vi "Register gRPC Messages.vi"(8 "error in (no error)":errorcluster, 11 "Template Server in":refnum<class "HVC5.lvclass">) -> (0 "error out":errorcluster, 3 "Template Server out":refnum<class "HVC5.lvclass">)   [LabVIEW 2019, in "HVC5.lvlib" / "HVC5.lvclass"]
uses:
  HVC5.lvclass
  gRPC lvSupport/Server API/typeDefs/Message Metadata.ctl
  gRPC lvSupport/Server API/typeDefs/Message Element Metadata.ctl
  gRPC lvSupport/Server API/typeDefs/Message Element Type.ctl
  HVC5.lvclass/HVC5.ctl
  gRPC lvSupport/gprc-lvsupport.lvlib
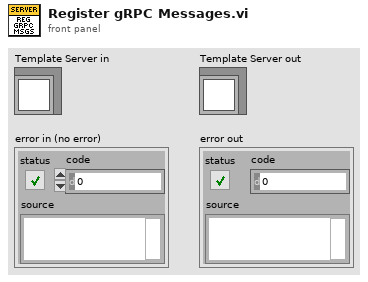
[diagram p1: front panel]
types:
  T1 = typedef "HVC5.lvlib/gprc-lvsupport.lvlib/Message Metadata.ctl" = cluster{"Name":string, "Elements":T2[]}
  T2 = typedef "HVC5.lvlib/gprc-lvsupport.lvlib/Message Element Metadata.ctl" = cluster{"Embedded Message Name":string, "Protobuf Index":i32, "MessageElementType":T3, "Repeated":bool}
  T3 = typedef "HVC5.lvlib/gprc-lvsupport.lvlib/Message Element Type.ctl" = enum32{"Int32Value", "FloatValue", "DoubleValue", "BoolValue", "StringValue", "MessageValue", "Int64Value", "UInt32Value", "UInt64Value", "EnumValue"}
  T4 = typedef "HVC5.lvlib/gprc-lvsupport.lvlib/grpcId.ctl" = u64
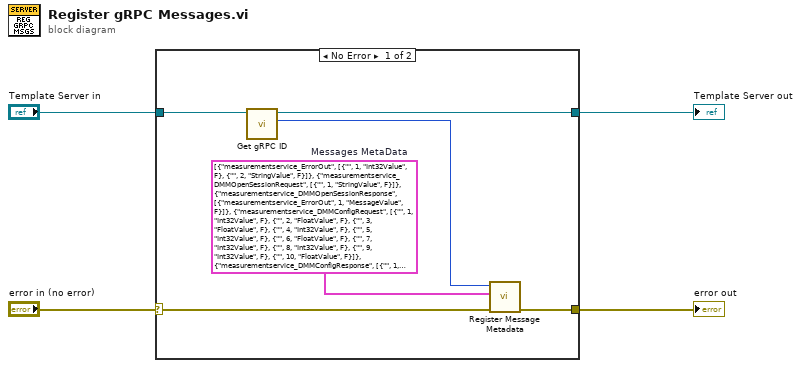
[diagram p0: block diagram]
diagram:
  n1 = case shown="No Error" "error in (no error)" {
    selector: "error in (no error)" -> [w5 w12]
    tunnel: [w10 w11] -> w4
    tunnel: [w9 w12] -> w3
    tunnel: "Template Server in" -> [w7 w11]
    frame No Error {
      w6 = T1[] [{"Name"="measurementservice_ErrorOut", "Elements"=[{"Embedded Message Name"="", "Protobuf Index"=1, "MessageElementType"=enum."Int32Value", "Repeated"=FALSE}, {"Embedded Message Name"="", "Protobuf Index"=2, "MessageElementType"=enum."StringValue", "Repeated"=FALSE}]}, {"Name"="measurementservice_DMMOpenSessionRequest", "Elements"=[{"Embedded Message Name"="", "Protobuf Index"=1, "MessageElementType"=enum."StringValue", "Repeated"=FALSE}]}, {"Name"="measurementservice_DMMOpenSessionResponse", "Elements"=[{"Embedded Message Name"="measurementservice_ErrorOut", "Protobuf Index"=1, "MessageElementType"=enum."MessageValue", "Repeated"=FALSE}]}, {"Name"="measurementservice_DMMConfigRequest", "Elements"=[{"Embedded Message Name"="", "Protobuf Index"=1, "MessageElementType"=enum."Int32Value", "Repeated"=FALSE}, {"Embedded Message Name"="", "Protobuf Index"=2, "MessageElementType"=enum."FloatValue", "Repeated"=FALSE}, {"Embedded Message Name"="", "Protobuf Index"=3, "MessageElementType"=enum."FloatValue", "Repeated"=FALSE}, {"Embedded Message Name"="", "Protobuf Index"=4, "MessageElementType"=enum."Int32Value", "Repeated"=FALSE}, {"Embedded Message Name"="", "Protobuf Index"=5, "MessageElementType"=enum."Int32Value", "Repeated"=FALSE}, {"Embedded Message Name"="", "Protobuf Index"=6, "MessageElementType"=enum."FloatValue", "Repeated"=FALSE}, {"Embedded Message Name"="", "Protobuf Index"=7, "MessageElementType"=enum."Int32Value", "Repeated"=FALSE}, {"Embedded Message Name"="", "Protobuf Index"=8, "MessageElementType"=enum."Int32Value", "Repeated"=FALSE}, {"Embedded Message Name"="", "Protobuf Index"=9, "MessageElementType"=enum."Int32Value", "Repeated"=FALSE}, {"Embedded Message Name"="", "Protobuf Index"=10, "MessageElementType"=enum."FloatValue", "Repeated"=FALSE}]}, {"Name"="measurementservice_DMMConfigResponse", "Elements"=[{"Embedded Message Name"="", "Protobuf Index"=1, "MessageElementType"=enum."Int32Value", "Repeated"=FALSE}, {"Embedded Message Name"="", "Protobuf Index"=2, "MessageElementType"=enum."FloatValue", "Repeated"=FALSE}, {"Embedded Message Name"="", "Protobuf Index"=3, "MessageElementType"=enum."FloatValue", "Repeated"=FALSE}, {"Embedded Message Name"="", "Protobuf Index"=4, "MessageElementType"=enum."Int32Value", "Repeated"=FALSE}, {"Embedded Message Name"="", "Protobuf Index"=5, "MessageElementType"=enum."Int32Value", "Repeated"=FALSE}, {"Embedded Message Name"="", "Protobuf Index"=6, "MessageElementType"=enum."FloatValue", "Repeated"=FALSE}, {"Embedded Message Name"="", "Protobuf Index"=7, "MessageElementType"=enum."Int32Value", "Repeated"=FALSE}, {"Embedded Message Name"="", "Protobuf Index"=8, "MessageElementType"=enum."Int32Value", "Repeated"=FALSE}, {"Embedded Message Name"="", "Protobuf Index"=9, "MessageElementType"=enum."Int32Value", "Repeated"=FALSE}, {"Embedded Message Name"="", "Protobuf Index"=10, "MessageElementType"=enum."FloatValue", "Repeated"=FALSE}, {"Embedded Message Name"="measurementservice_ErrorOut", "Protobuf Index"=11, "MessageElementType"=enum."MessageValue", "Repeated"=FALSE}]}, {"Name"="measurementservice_DMMVoltageRequest", "Elements"=[]}, {"Name"="measurementservice_DMMVoltageData", "Elements"=[{"Embedded Message Name"="", "Protobuf Index"=1, "MessageElementType"=enum."FloatValue", "Repeated"=TRUE}, {"Embedded Message Name"="measurementservice_ErrorOut", "Protobuf Index"=2, "MessageElementType"=enum."MessageValue", "Repeated"=FALSE}]}, {"Name"="measurementservice_DMMCloseSessionRequest", "Elements"=[]}, {"Name"="measurementservice_DMMCloseSessionResponse", "Elements"=[{"Embedded Message Name"="measurementservice_ErrorOut", "Protobuf Index"=1, "MessageElementType"=enum."MessageValue", "Repeated"=FALSE}]}, {"Name"="measurementservice_DMMSelfCalRequest", "Elements"=[{"Embedded Message Name"="", "Protobuf Index"=1, "MessageElementType"=enum."StringValue", "Repeated"=FALSE}]}, {"Name"="measurementservice_DMMSelfCalResponse", "Elements"=[{"Embedded Message Name"="measurementservice_ErrorOut", "Protobuf Index"=1, "MessageElementType"=enum."MessageValue", "Repeated"=FALSE}]}, {"Name"="measurementservice_DMMResetRequest", "Elements"=[{"Embedded Message Name"="", "Protobuf Index"=1, "MessageElementType"=enum."StringValue", "Repeated"=FALSE}]}, {"Name"="measurementservice_DMMResetResponse", "Elements"=[{"Embedded Message Name"="measurementservice_ErrorOut", "Protobuf Index"=1, "MessageElementType"=enum."MessageValue", "Repeated"=FALSE}]}, {"Name"="measurementservice_SMUOpenSessionRequest", "Elements"=[{"Embedded Message Name"="", "Protobuf Index"=1, "MessageElementType"=enum."StringValue", "Repeated"=FALSE}]}, {"Name"="measurementservice_SMUOpenSessionResponse", "Elements"=[{"Embedded Message Name"="measurementservice_ErrorOut", "Protobuf Index"=1, "MessageElementType"=enum."MessageValue", "Repeated"=FALSE}]}, {"Name"="measurementservice_SMUConfigRequest", "Elements"=[{"Embedded Message Name"="", "Protobuf Index"=1, "MessageElementType"=enum."StringValue", "Repeated"=FALSE}, {"Embedded Message Name"="", "Protobuf Index"=2, "MessageElementType"=enum."Int32Value", "Repeated"=FALSE}, {"Embedded Message Name"="", "Protobuf Index"=3, "MessageElementType"=enum."Int32Value", "Repeated"=FALSE}, {"Embedded Message Name"="", "Protobuf Index"=4, "MessageElementType"=enum."Int32Value", "Repeated"=FALSE}, {"Embedded Message Name"="", "Protobuf Index"=5, "MessageElementType"=enum."FloatValue", "Repeated"=FALSE}, {"Embedded Message Name"="", "Protobuf Index"=6, "MessageElementType"=enum."FloatValue", "Repeated"=FALSE}, {"Embedded Message Name"="", "Protobuf Index"=7, "MessageElementType"=enum."Int32Value", "Repeated"=FALSE}, {"Embedded Message Name"="", "Protobuf Index"=8, "MessageElementType"=enum."Int32Value", "Repeated"=FALSE}, {"Embedded Message Name"="", "Protobuf Index"=9, "MessageElementType"=enum."FloatValue", "Repeated"=FALSE}, {"Embedded Message Name"="", "Protobuf Index"=10, "MessageElementType"=enum."FloatValue", "Repeated"=FALSE}, {"Embedded Message Name"="", "Protobuf Index"=11, "MessageElementType"=enum."FloatValue", "Repeated"=FALSE}, {"Embedded Message Name"="", "Protobuf Index"=12, "MessageElementType"=enum."Int32Value", "Repeated"=FALSE}]}, {"Name"="measurementservice_SMUConfigResponse", "Elements"=[{"Embedded Message Name"="", "Protobuf Index"=1, "MessageElementType"=enum."StringValue", "Repeated"=FALSE}, {"Embedded Message Name"="", "Protobuf Index"=2, "MessageElementType"=enum."Int32Value", "Repeated"=FALSE}, {"Embedded Message Name"="", "Protobuf Index"=3, "MessageElementType"=enum."Int32Value", "Repeated"=FALSE}, {"Embedded Message Name"="", "Protobuf Index"=4, "MessageElementType"=enum."Int32Value", "Repeated"=FALSE}, {"Embedded Message Name"="", "Protobuf Index"=5, "MessageElementType"=enum."FloatValue", "Repeated"=FALSE}, {"Embedded Message Name"="", "Protobuf Index"=6, "MessageElementType"=enum."FloatValue", "Repeated"=FALSE}, {"Embedded Message Name"="", "Protobuf Index"=7, "MessageElementType"=enum."Int32Value", "Repeated"=FALSE}, {"Embedded Message Name"="", "Protobuf Index"=8, "MessageElementType"=enum."Int32Value", "Repeated"=FALSE}, {"Embedded Message Name"="", "Protobuf Index"=9, "MessageElementType"=enum."FloatValue", "Repeated"=FALSE}, {"Embedded Message Name"="", "Protobuf Index"=10, "MessageElementType"=enum."FloatValue", "Repeated"=FALSE}, {"Embedded Message Name"="", "Protobuf Index"=11, "MessageElementType"=enum."FloatValue", "Repeated"=FALSE}, {"Embedded Message Name"="", "Protobuf Index"=12, "MessageElementType"=enum."Int32Value", "Repeated"=FALSE}, {"Embedded Message Name"="measurementservice_ErrorOut", "Protobuf Index"=13, "MessageElementType"=enum."MessageValue", "Repeated"=FALSE}]}, {"Name"="measurementservice_SMUEnableRequest", "Elements"=[]}, {"Name"="measurementservice_SMUEnableResponse", "Elements"=[{"Embedded Message Name"="measurementservice_ErrorOut", "Protobuf Index"=1, "MessageElementType"=enum."MessageValue", "Repeated"=FALSE}]}, {"Name"="measurementservice_SMUDisableRequest", "Elements"=[]}, {"Name"="measurementservice_SMUDisableResponse", "Elements"=[{"Embedded Message Name"="measurementservice_ErrorOut", "Protobuf Index"=1, "MessageElementType"=enum."MessageValue", "Repeated"=FALSE}]}, {"Name"="measurementservice_SMUCurrentRequest", "Elements"=[]}, {"Name"="measurementservice_SMUCurrentData", "Elements"=[{"Embedded Message Name"="", "Protobuf Index"=1, "MessageElementType"=enum."FloatValue", "Repeated"=FALSE}, {"Embedded Message Name"="measurementservice_ErrorOut", "Protobuf Index"=2, "MessageElementType"=enum."MessageValue", "Repeated"=FALSE}]}, {"Name"="measurementservice_SMUCloseSessionRequest", "Elements"=[]}, {"Name"="measurementservice_SMUCloseSessionResponse", "Elements"=[{"Embedded Message Name"="measurementservice_ErrorOut", "Protobuf Index"=1, "MessageElementType"=enum."MessageValue", "Repeated"=FALSE}]}, {"Name"="measurementservice_SMUSelfCalRequest", "Elements"=[{"Embedded Message Name"="", "Protobuf Index"=1, "MessageElementType"=enum."StringValue", "Repeated"=FALSE}]}, {"Name"="measurementservice_SMUSelfCalResponse", "Elements"=[{"Embedded Message Name"="measurementservice_ErrorOut", "Protobuf Index"=1, "MessageElementType"=enum."MessageValue", "Repeated"=FALSE}]}, {"Name"="measurementservice_SMUResetRequest", "Elements"=[{"Embedded Message Name"="", "Protobuf Index"=1, "MessageElementType"=enum."StringValue", "Repeated"=FALSE}]}, {"Name"="measurementservice_SMUResetResponse", "Elements"=[{"Embedded Message Name"="measurementservice_ErrorOut", "Protobuf Index"=1, "MessageElementType"=enum."MessageValue", "Repeated"=FALSE}]}, {"Name"="measurementservice_NI2576MUXOpenSessionRequest", "Elements"=[{"Embedded Message Name"="", "Protobuf Index"=1, "MessageElementType"=enum."StringValue", "Repeated"=FALSE}, {"Embedded Message Name"="", "Protobuf Index"=2, "MessageElementType"=enum."StringValue", "Repeated"=FALSE}]}, {"Name"="measurementservice_NI2576MUXOpenSessionResponse", "Elements"=[{"Embedded Message Name"="measurementservice_ErrorOut", "Protobuf Index"=1, "MessageElementType"=enum."MessageValue", "Repeated"=FALSE}]}, {"Name"="measurementservice_NI2576MUXCloseChannelRequest", "Elements"=[{"Embedded Message Name"="", "Protobuf Index"=1, "MessageElementType"=enum."StringValue", "Repeated"=FALSE}, {"Embedded Message Name"="", "Protobuf Index"=2, "MessageElementType"=enum."StringValue", "Repeated"=FALSE}]}, {"Name"="measurementservice_NI2576MUXCloseChannelResponse", "Elements"=[{"Embedded Message Name"="measurementservice_ErrorOut", "Protobuf Index"=1, "MessageElementType"=enum."MessageValue", "Repeated"=FALSE}]}, {"Name"="measurementservice_NI2576MUXOpenChannelRequest", "Elements"=[{"Embedded Message Name"="", "Protobuf Index"=1, "MessageElementType"=enum."StringValue", "Repeated"=FALSE}, {"Embedded Message Name"="", "Protobuf Index"=2, "MessageElementType"=enum."StringValue", "Repeated"=FALSE}]}, {"Name"="measurementservice_NI2576MUXOpenChannelResponse", "Elements"=[{"Embedded Message Name"="measurementservice_ErrorOut", "Protobuf Index"=1, "MessageElementType"=enum."MessageValue", "Repeated"=FALSE}]}, {"Name"="measurementservice_NI2576MUXDisconnectAllRequest", "Elements"=[]}, {"Name"="measurementservice_NI2576MUXDisconnectAllResponse", "Elements"=[{"Embedded Message Name"="measurementservice_ErrorOut", "Protobuf Index"=1, "MessageElementType"=enum."MessageValue", "Repeated"=FALSE}]}, {"Name"="measurementservice_NI2576MUXCloseSessionRequest", "Elements"=[]}, {"Name"="measurementservice_NI2576MUXCloseSessionResponse", "Elements"=[{"Embedded Message Name"="measurementservice_ErrorOut", "Protobuf Index"=1, "MessageElementType"=enum."MessageValue", "Repeated"=FALSE}]}, {"Name"="measurementservice_NI2576MUXResetRequest", "Elements"=[{"Embedded Message Name"="", "Protobuf Index"=1, "MessageElementType"=enum."StringValue", "Repeated"=FALSE}]}, {"Name"="measurementservice_NI2576MUXResetResponse", "Elements"=[{"Embedded Message Name"="measurementservice_ErrorOut", "Protobuf Index"=1, "MessageElementType"=enum."MessageValue", "Repeated"=FALSE}]}, {"Name"="measurementservice_InvokeRequest", "Elements"=[{"Embedded Message Name"="", "Protobuf Index"=1, "MessageElementType"=enum."StringValue", "Repeated"=FALSE}, {"Embedded Message Name"="", "Protobuf Index"=2, "MessageElementType"=enum."StringValue", "Repeated"=FALSE}]}, {"Name"="measurementservice_InvokeResponse", "Elements"=[{"Embedded Message Name"="", "Protobuf Index"=1, "MessageElementType"=enum."Int32Value", "Repeated"=FALSE}]}, {"Name"="measurementservice_QueryRequest", "Elements"=[{"Embedded Message Name"="", "Protobuf Index"=1, "MessageElementType"=enum."StringValue", "Repeated"=FALSE}]}, {"Name"="measurementservice_QueryResponse", "Elements"=[{"Embedded Message Name"="", "Protobuf Index"=1, "MessageElementType"=enum."StringValue", "Repeated"=FALSE}, {"Embedded Message Name"="", "Protobuf Index"=2, "MessageElementType"=enum."Int32Value", "Repeated"=FALSE}]}, {"Name"="measurementservice_RegistrationRequest", "Elements"=[{"Embedded Message Name"="", "Protobuf Index"=1, "MessageElementType"=enum."StringValue", "Repeated"=FALSE}]}, {"Name"="measurementservice_ServerEvent", "Elements"=[{"Embedded Message Name"="", "Protobuf Index"=1, "MessageElementType"=enum."StringValue", "Repeated"=FALSE}, {"Embedded Message Name"="", "Protobuf Index"=2, "MessageElementType"=enum."Int32Value", "Repeated"=FALSE}, {"Embedded Message Name"="", "Protobuf Index"=3, "MessageElementType"=enum."Int32Value", "Repeated"=FALSE}]}]  # Messages MetaData
      n2 = call "Get gRPC ID.vi"("OOP Server in"=w7) -> ("gRPC ID"=w8:T4, "OOP Server out"=w10:refnum<class "HVC5.lvclass">)  [unwired: 9 in]
      n3 = call "Register Message Metadata.vi"("error in (no error)"=w5, "Messages"=w6, "gRPCid"=w8) -> ("error out"=w9:errorcluster)  [unwired: 7 in, 1 out]
    }
    frame Error {
    }
  }
  "Template Server out" <- w4
  "error out" <- w3
